vi "Send coord.vi"(8 "error in (no error)":errorcluster, 9 "x":dbl, 10 "y":dbl, 11 "connection ID":refnum<k16>) -> (0 "error out":errorcluster, 2 "Engine":dbl, 3 "connection ID out":refnum<k16>)   [LabVIEW 2020]
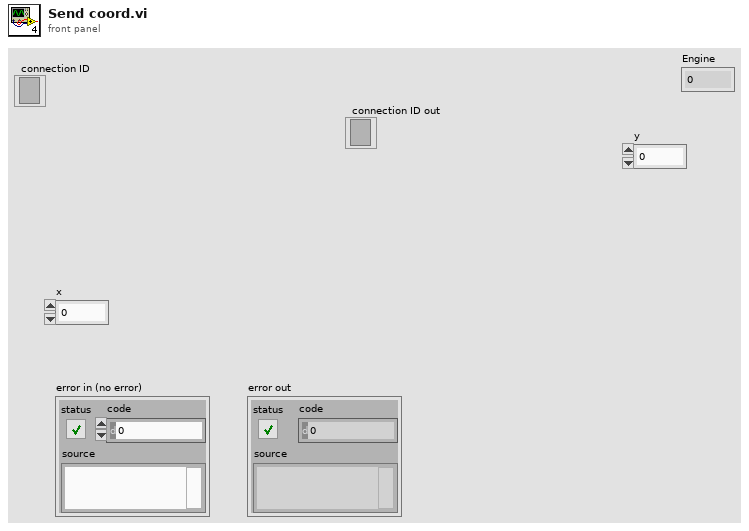
[diagram p1: front panel]
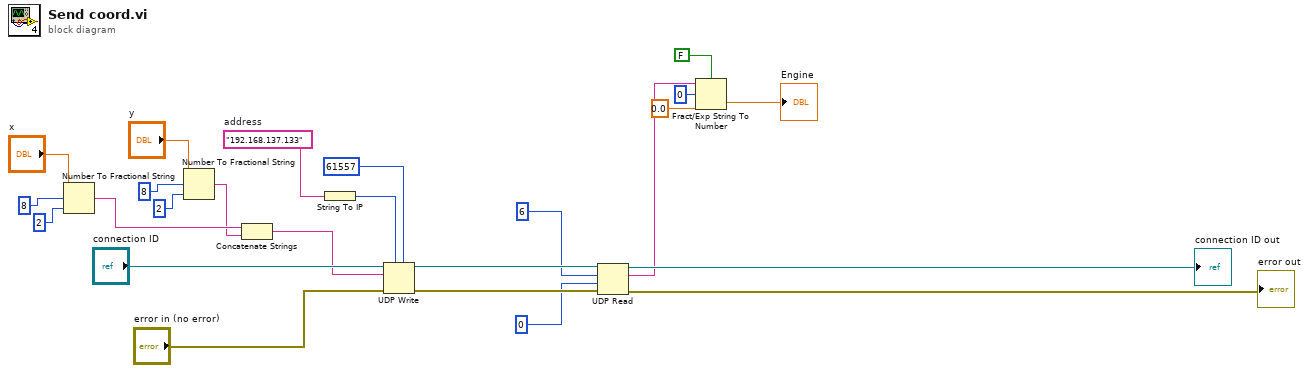
[diagram p0: block diagram]
diagram:
  w17 = "192.168.137.133"  # address
  n1 = Number To Fractional String(number="x", width (-)=i16 8, precision (6)=i16 2) -> (F-format string=w14:string)  [unwired: 1 in]
  n2 = Number To Fractional String(number="y", width (-)=i16 8, precision (6)=i16 2) -> (F-format string=w13:string)  [unwired: 1 in]
  n3 = Concatenate Strings(w14, w13) -> (w12:string)
  n4 = String To IP(1:w17) -> (0:w16:u32)
  n5 = UDP Write(address=w16, port or service name=u16 61557, connection ID="connection ID", data in=w12, 8:"error in (no error)") -> (error out=w10:errorcluster, 3:w11:refnum<k16>)  [unwired: 1 in]
  n6 = UDP Read(connection ID=w11, max size (548)=6, timeout ms (25000)=0, 8:w10) -> (data out=w2:string, error out=→"error out":errorcluster, 3:→"connection ID out":refnum<k16>)  [unwired: 2 out]
  n7 = Fract/Exp String To Number(use system decimal point (T)=FALSE, string=w2, offset=0, default (0 dbl)=0.0 ("default (0 DBL)")) -> (number=→"Engine":dbl)  [unwired: 1 out]
